vi "if_v0_v1.vi"() -> ()   [LabVIEW 2009]
panel:
  out "Rez":dbl
  in  "B":dbl
  in  "A":dbl
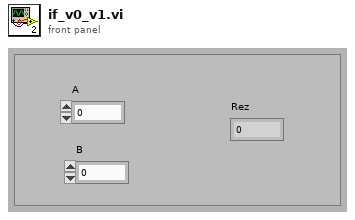
[diagram p1: front panel]
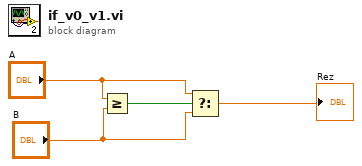
[diagram p0: block diagram]
diagram:
  n1 = Greater Or Equal?(x="A", y="B") -> (x >= y?=w4:bool)
  n2 = Select(t="A", s=w4, f="B") -> (s? t:f=→"Rez":dbl)
